vi "Ramp Actuator Speed.vi"(7 "Up to Down":bool, 8 "error in (no error)":errorcluster, 9 "RA Down Volt":dbl, 10 "RA Up Volt":dbl, 11 "AIDeviceRef":T1) -> (2 "Ramp Actuator Ouput":dbl)   [LabVIEW 2011]
uses:
  <vilib>/Rock Robotics/WPI/AnalogChannel/WPI_AnalogChannelDevRef.ctl
  <vilib>/Rock Robotics/SystemInterfaces/Typedef/FPGA_TypedefAnalogModule.ctl
  <vilib>/Rock Robotics/SystemInterfaces/AI/FPGA_AIChannel.ctl
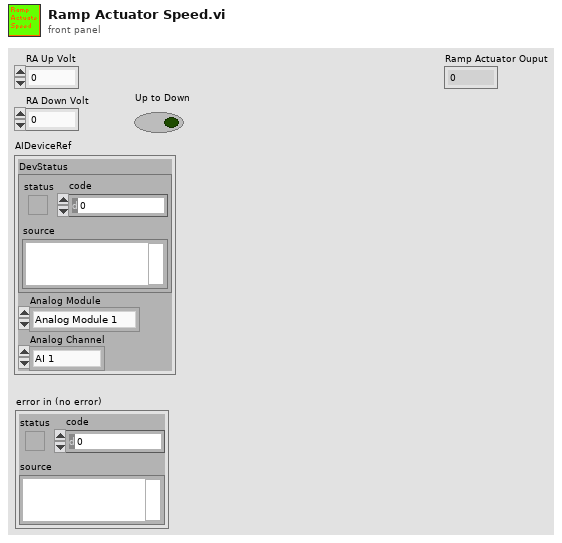
[diagram p1: front panel]
types:
  T1 = typedef "WPI_AnalogChannelDevRef.ctl" = cluster{"DevStatus":errorcluster, "Analog Module":T2, "Analog Channel":T3}
  T2 = typedef "FPGA_TypedefAnalogModule.ctl" = enum16{"Analog Module 1", "Analog Module 2"}
  T3 = typedef "FPGA_AIChannel.ctl" = enum8{"AI 1", "AI 2", "AI 3", "AI 4", "AI 5", "AI 6", "AI 7", "AI 8", "Invalid"}
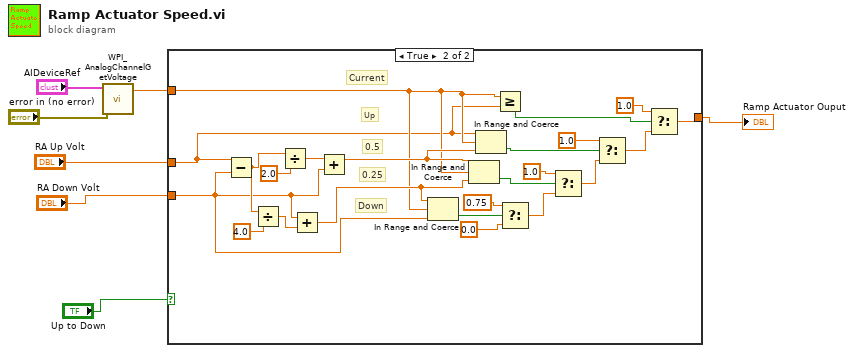
[diagram p0: block diagram]
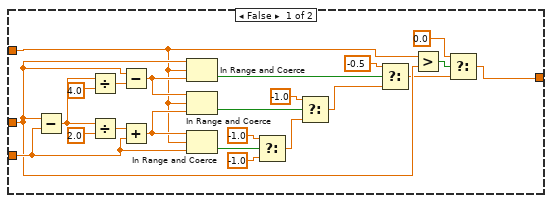
[diagram p2: hidden frame]
diagram:
  n1 = call <vilib>:"WPI_AnalogChannelGetVoltage.vi"("error in (no error)"="error in (no error)", "AIDeviceRef"="AIDeviceRef") -> ("Voltage"=w4:dbl)  [unwired: 7 in, 2 out]
  n2 = case shown="True" "Up to Down" {
    tunnel: "RA Down Volt" -> [w25 w37]
    tunnel: w4 -> [w8 w36]
    tunnel: "RA Up Volt" -> [w13 w35]
    tunnel: [w9 w31] -> w1
    frame False {
      n3 = Subtract(x=w13, y=w25) -> (x-y=w28:dbl)
      n4 = Divide(x=w28, y=4.0) -> (x/y=w26:dbl)
      n5 = Divide(x=w28, y=2.0) -> (x/y=w29:dbl)
      n6 = Subtract(x=w13, y=w26) -> (x-y=w15:dbl)
      n7 = Add(x=w29, y=w25) -> (x+y=w17:dbl)
      n8 = In Range and Coerce(upper limit=w13, x=w8, lower limit=w15) -> (In Range?=w14:bool)  [unwired: 1 out]
      n9 = In Range and Coerce(upper limit=w15, x=w8, lower limit=w17) -> (In Range?=w16:bool)  [unwired: 1 out]
      n10 = In Range and Coerce(upper limit=w17, x=w8, lower limit=w25) -> (In Range?=w24:bool)  [unwired: 1 out]
      n11 = Select(t=-1.0, s=w24, f=-1.0) -> (s? t:f=w21:dbl)
      n12 = Select(t=-1.0, s=w16, f=w21) -> (s? t:f=w19:dbl)
      n13 = Select(t=-0.5, s=w14, f=w19) -> (s? t:f=w12:dbl)
      n14 = Greater?(x=w8, y=w13) -> (0:w11:bool)
      n15 = Select(t=0.0, s=w11, f=w12) -> (s? t:f=w9:dbl)
    }
    frame True {
      # "Current"
      # "Down"
      # "0.25"
      # "0.5"
      # "Up"
      n16 = Subtract(x=w35, y=w37) -> (x-y=w50:dbl)
      n17 = Divide(x=w50, y=4.0) -> (x/y=w49:dbl)
      n18 = Divide(x=w50, y=2.0) -> (x/y=w51:dbl)
      n19 = Add(x=w37, y=w49) -> (x+y=w39:dbl)
      n20 = Add(x=w51, y=w37) -> (x+y=w38:dbl)
      n21 = In Range and Coerce(upper limit=w39, x=w36, lower limit=w37) -> (In Range?=w41:bool)  [unwired: 1 out]
      n22 = In Range and Coerce(upper limit=w38, x=w36, lower limit=w39) -> (In Range?=w45:bool)  [unwired: 1 out]
      n23 = In Range and Coerce(upper limit=w35, x=w36, lower limit=w38) -> (In Range?=w40:bool)  [unwired: 1 out]
      n24 = Greater Or Equal?(x=w36, y=w35) -> (x >= y?=w34:bool)
      n25 = Select(t=0.75, s=w41, f=0.0) -> (s? t:f=w44:dbl)
      n26 = Select(t=1.0, s=w45, f=w44) -> (s? t:f=w47:dbl)
      n27 = Select(t=1.0, s=w40, f=w47) -> (s? t:f=w32:dbl)
      n28 = Select(t=1.0, s=w34, f=w32) -> (s? t:f=w31:dbl)
    }
  }
  "Ramp Actuator Ouput" <- w1
